vi "K_S30_VISA F101.vi"(5 "Index":u8, 6 "error in":errorcluster, 7 "Dialog":bool=TRUE, 8 "Parameter 0 .. 4":u8[](array[numeric]), 9 "Dev Addr":u8=250) -> (0 "error out":errorcluster, 2 "Org. Parameter 0 .. 4":u8[](array[numeric]))   [LabVIEW 2012]
panel:
  # "Function101: Write a single configurtion byte, using funtion 100\n\nWarning!\n\nPlease be careful, using this function! \nWrong configuration changes the function of the device! \nMake sure that you save first the origignal configuration with function 100.\nIf your device supports F32 (5.20-4.1 and earlier), then use F33 instead of this function.\n\nusing VISA\nKeller AG für Druckmesstechnik, 29.5.08 b.v."
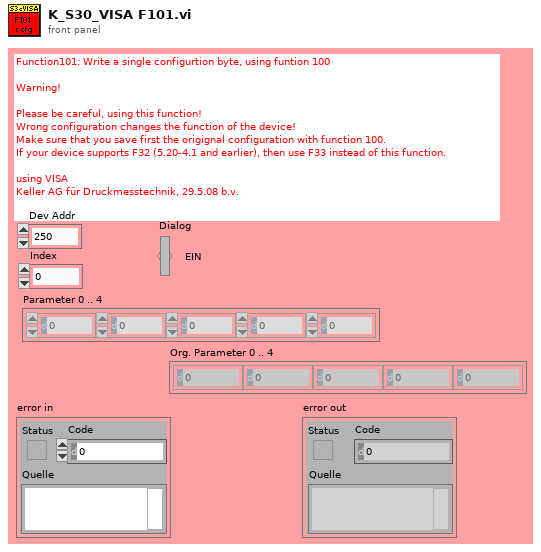
[diagram p1: front panel]
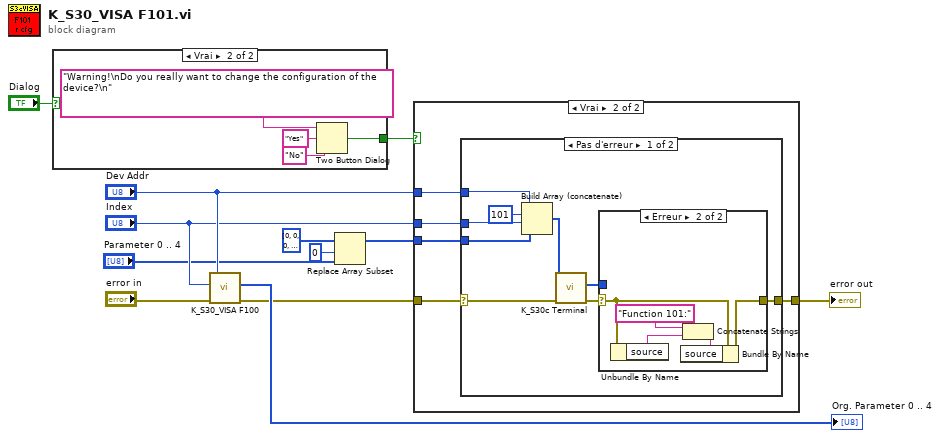
[diagram p0: block diagram]
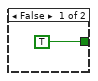
[diagram p2: hidden frame]
diagram:
  n1 = case shown="Vrai" "Dialog" {
    tunnel: [TRUE w14] -> w6
    frame False {
    }
    frame True {
      n2 = Two Button Dialog(message="Warning!\nDo you really want to change the configuration of the device?\n" ("Nachricht"), 1:"No" ("F-Schaltflächenname (\"Abbrechen\")"), 2:"Yes" ("T-Schaltflächenname (\"OK\")")) -> (T button?=w14:bool)
    }
  }
  n3 = call "K_S30_VISA F100.vi"("error in"="error in", "Index"="Index", "Address"="Dev Addr") -> ("error out"=w8:errorcluster, "para 0..4"=→"Org. Parameter 0 .. 4":u8[])  [unwired: 3 in]
  n4 = Replace Array Subset(array=i32[] [0, 0, 0, 0, 0], new element="Parameter 0 .. 4", index=0 ("Index")) -> (w1:i32[])
  n5 = case shown="Vrai" w6 {
    tunnel: [w18 w23] -> w12
    tunnel: "Dev Addr" -> [_ w22]
    tunnel: "Index" -> [_ w21]
    tunnel: w8 -> [w18 w20]
    tunnel: w1 -> [_ w19]
    frame False {
    }
    frame True {
      n6 = case shown="Pas d'erreur" w20 {
        selector: w20 -> [w30 w39]
        tunnel: [w26 w39] -> w23
        tunnel: w22 -> [w29 _]
        tunnel: w21 -> [w28 _]
        tunnel: w19 -> [w27 _]
        frame No Error {
          n7 = Build Array (concatenate)(w29, u8 101 ("Element"), w28, w27) -> (w31:i32[])
          n8 = call "K_S30c Terminal.vi"("error in"=w30, "request"=w31) -> ("error out"=w25:errorcluster, "response"=w24:u8[])  [unwired: 4 in]
          n9 = case shown="Erreur" w25 {
            selector: w25 -> [w33 w38]
            tunnel: [w33 w36] -> w26
            tunnel: w24 -> [_ _]
            frame No Error {
            }
            frame Error {
              n10 = Unbundle By Name(w38) -> ("source"=w35:string)
              n11 = Concatenate Strings("Function 101:" ("String"), w35) -> (w37:string)
              n12 = Bundle By Name(cluster=w38, "source"=w37) -> (w36:errorcluster)
            }
          }
        }
        frame Error {
        }
      }
    }
  }
  "error out" <- w12
